vi "Demo.vi"() -> ()   [LabVIEW 2021]
doc: "本VI是为《我和LabVIEW》一书编写的示例。\n关于本书的介绍请参考网页：\nhttp://ruanqizhen.spaces.live.com/blog/cns!5852D4F797C53FB6!4310.entry"
panel:
  out "结果":refnum<class "基本数据类型.lvclass">[](array[class])
  out "结果":refnum<class "簇类型.lvclass">
  out "结果":refnum<class "数值类型.lvclass">
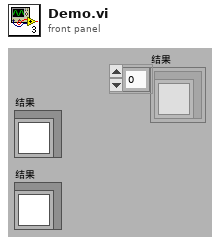
[diagram p1: front panel]
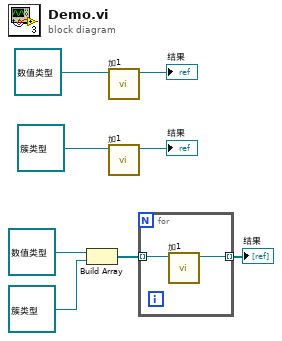
[diagram p0: block diagram]
diagram:
  n1 = Build Array(refnum<class "数值类型.lvclass"> refnum ("数值类型.lvclass"), refnum<class "簇类型.lvclass"> refnum ("簇类型.lvclass")) -> (w2:refnum<class "基本数据类型.lvclass">[])
  n2 = call "加1.vi"("基本数据类型 in"=refnum<class "数值类型.lvclass"> refnum ("数值类型.lvclass")) -> ("基本数据类型 out"=→"结果":refnum<class "数值类型.lvclass">)  [unwired: 1 in, 9 out]
  n3 = call "加1.vi"("基本数据类型 in"=refnum<class "簇类型.lvclass"> refnum ("簇类型.lvclass")) -> ("基本数据类型 out"=→"结果":refnum<class "簇类型.lvclass">)  [unwired: 1 in, 9 out]
  n4 = for {
    tunnel: w2 -> [w10] mode=indexing
    tunnel: [w9] -> w1 mode=indexing
    n5 = call "加1.vi"("基本数据类型 in"=w10) -> ("基本数据类型 out"=w9:refnum<class "基本数据类型.lvclass">)  [unwired: 1 in, 9 out]
  }
  "结果" <- w1
